vi "Display_LDA_data_rate.vi"(1 "Hydrosonic Setting %":dbl, 2 "Current Sampling Freq (Hz)":dbl format="%#.0f") -> ()   [LabVIEW 2011]
panel:
  out "Waveform Chart":T1(graph)
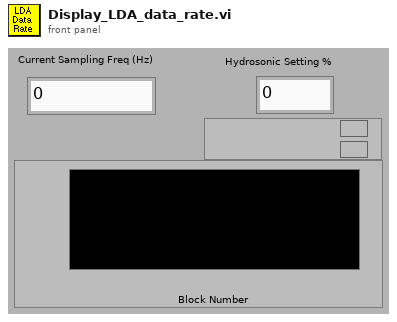
[diagram p1: front panel]
types:
  T1 = cluster{"Hydrosonic Setting %":dbl, "Current Sampling Freq (Hz)":dbl}
  T2 = cluster{"Current Sampling Freq (Hz)":dbl, "Hydrosonic Setting %":dbl}
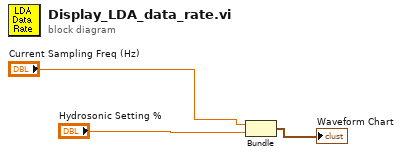
[diagram p0: block diagram]
diagram:
  n1 = Bundle("Current Sampling Freq (Hz)"="Current Sampling Freq (Hz)", "Hydrosonic Setting %"="Hydrosonic Setting %") -> (→"Waveform Chart":T2)  [unwired: 1 out]
